vi "Format Relative Time.vi"(4 "Unix ns":i64) -> (7 "String":string)   [LabVIEW 2020, in "VolatusSeqGUI.lvlib" / "Sequencing Control.lvclass"]
uses:
  Sequencing Control.lvclass
  Sequencing Control.lvclass/Sequencing Control.ctl
  lv-vecto/Vecto/Vecto.lvlib
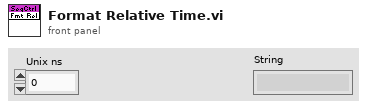
[diagram p1: front panel]
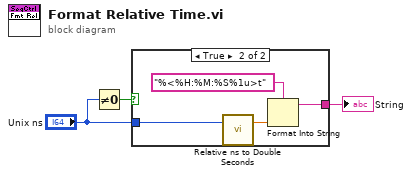
[diagram p0: block diagram]
diagram:
  n1 = Not Equal To 0?(x="Unix ns") -> (x != 0?=w1:bool)
  n2 = case shown="True" w1 {
    tunnel: [_ w5] -> w3
    tunnel: "Unix ns" -> [_ w4]
    frame False {
    }
    frame True {
      n3 = call "Relative ns to Double Seconds.vi"("relative ns"=w4) -> ("Double s"=w6:dbl)  [unwired: 6 in]
      n4 = Format Into String(format string="%<%H:%M:%S%1u>t", w6) -> (resulting string=w5:string)  [unwired: 2 in, 1 out]
    }
  }
  "String" <- w3
